vi "(Sub) Read CMD Chack.vi"(8 "error in (no error)":errorcluster caption="에러 입력(에러 없음)", 10 "Read Data":string, 11 "Write CMD":string) -> (0 "error out":errorcluster caption="에러 출력", 2 "Read Success ?":bool, 3 "Data":string)   [LabVIEW 2017]
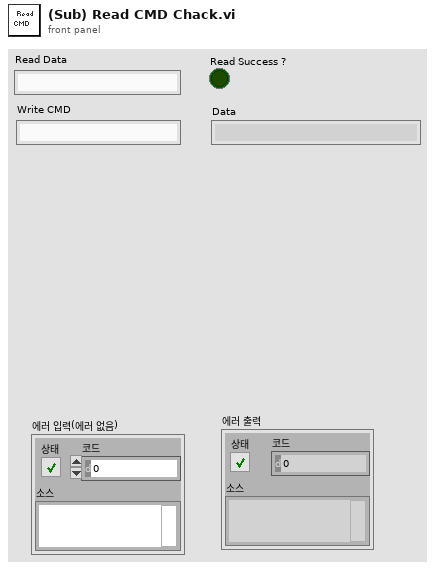
[diagram p1: front panel]
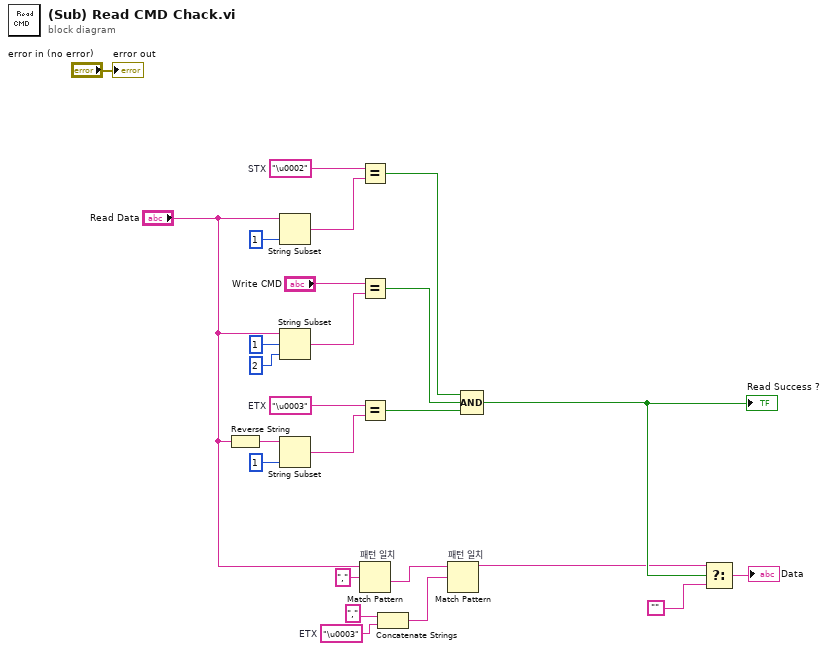
[diagram p0: block diagram]
diagram:
  w2 = "\u0003"  # ETX
  w21 = "\u0003"  # ETX
  w22 = "\u0002"  # STX
  n1 = Reverse String(1:"Read Data") -> (0:w25:string)
  n2 = String Subset(string="Read Data", length (rest)=1 ("길이(나머지)")) -> (substring=w23:string)  [unwired: 1 in]
  n3 = String Subset(string="Read Data", offset (0)=1 ("오프셋(0)"), length (rest)=2 ("길이(나머지)")) -> (substring=w18:string)
  n4 = String Subset(string=w25, length (rest)=1 ("길이(나머지)")) -> (substring=w24:string)  [unwired: 1 in]
  n5 = Equal?(x=w22, y=w23) -> (x = y?=w20:bool)
  n6 = Equal?(x="Write CMD", y=w18) -> (x = y?=w12:bool)
  n7 = Equal?(x=w21, y=w24) -> (x = y?=w11:bool)
  n8 = Match Pattern "패턴 일치"(string="Read Data", regular expression="," ("정규식")) -> (after substring=w4:string)  [unwired: 1 in, 3 out]
  n9 = Concatenate Strings("," ("정규식"), w2) -> (w1:string)
  n10 = Match Pattern "패턴 일치"(string=w4, regular expression=w1) -> (before substring=w7:string)  [unwired: 1 in, 3 out]
  n11 = Compound Arithmetic op=AND ("복합 연산")(w20, w12, w11) -> (w19:bool)
  "Read Success ?" <- w19
  n12 = Select(t=w7, s=w19, f="") -> (s? t:f=→"Data":string)
  "error out" <- "error in (no error)"
